vi "Driver Init.vi"(8 "error in (no error)":errorcluster, 11 "CAP-USB-1 in":refnum<class "CAP-USB-1.lvclass">) -> (0 "error out":errorcluster, 3 "CAP-USB-1 out":refnum<class "CAP-USB-1.lvclass">)   [LabVIEW 2014, in "CAP-USB-1.lvlib" / "CAP-USB-1.lvclass"]
doc: "Inicializa los valores de configuracion y diagnostico del Dispositivo"
uses:
  CAP-USB-1.lvclass
  CAP-USB-1.lvclass/CAP-USB-1.ctl
  DriverMasterSync/build/DriverMasterSync.lvlibp/Modules/HAL/DriverMasterSync/DriverMasterSyncClass/DriverMasterSync.lvclass
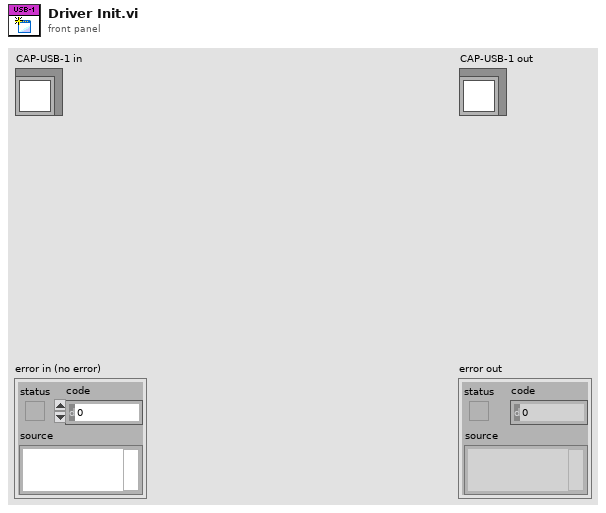
[diagram p1: front panel]
types:
  T1 = typedef "DriverMasterSync.lvlibp/HAL Config Data.ctl" = cluster{"HWSync Index":u32, "Driver Name":string, "Channel Mask":u64}
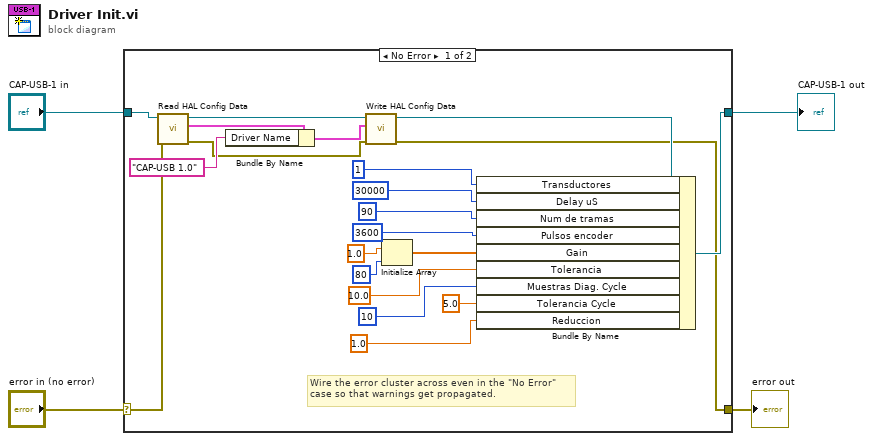
[diagram p0: block diagram]
diagram:
  n1 = case shown="No Error" "error in (no error)" {
    selector: "error in (no error)" -> [w8 w27]
    tunnel: [w7 w27] -> w3
    tunnel: [w25 w26] -> w1
    tunnel: "CAP-USB-1 in" -> [w15 w26]
    frame No Error {
      # "Wire the error cluster across even in the \"No Error\"\ncase so that warnings get propagated."
      n2 = call "Read HAL Config Data.vi"("error in (no error)"=w8, "DriverMasterSync in"=w15) -> ("error out"=w9:errorcluster, "HAL Config Data"=w14:T1, "DriverMasterSync out"=w11:refnum<class "CAP-USB-1.lvclass">)  [unwired: 7 in]
      n3 = Bundle By Name(cluster=w14, "Driver Name"="CAP-USB 1.0") -> (w12:T1)
      n4 = call "Write HAL Config Data.vi"("error in (no error)"=w9, "HAL Config Data"=w12, "DriverMasterSync in"=w11) -> ("error out"=w7:errorcluster, "DriverMasterSync out"=w10:refnum<class "CAP-USB-1.lvclass">)  [unwired: 7 in]
      n5 = Initialize Array(sgl 1.0 ("Offset"), 80 ("dimension size")) -> (w18:sgl[])
      n6 = Bundle By Name(cluster=w10, "Transductores"=u64 1 ("Config Data.Transductores"), "Delay uS"=30000 ("Config Data.Delay uS"), "Num de tramas"=u32 90 ("Config Data.Num de tramas"), "Pulsos encoder"=u16 3600 ("Config Data.Pulsos encoder"), "Gain"=w18, "Tolerancia"=sgl 10.0 ("Diagnostic Data.Tolerancia %"), "Muestras Diag. Cycle"=u32 10 ("Diagnostic Data.Muestras Diag. Cycle"), "Tolerancia Cycle"=sgl 5.0 ("Diagnostic Data.Tolerancia Cycle"), "Reduccion"=sgl 1.0 ("Diagnostic Data.Tolerancia %")) -> (w25:refnum<class "CAP-USB-1.lvclass">)
    }
    frame Error {
    }
  }
  "error out" <- w3
  "CAP-USB-1 out" <- w1
